vi "Harvest_Global.vi"() -> ()   [LabVIEW 2015]
panel:
  in  "stop":bool
  in  "Files pulled from Public":i32
  in  "Files Copied fr Server to Public":i32
  in  "Files copied fr Local to Public":i32
  in  "No Files to Pull":i32
  in  "Files pushed onto Server":i32
  in  "Done Transfer?":bool
  in  "No Files to Push":i32
  in  "File being transfered":path
  in  "Currently":string
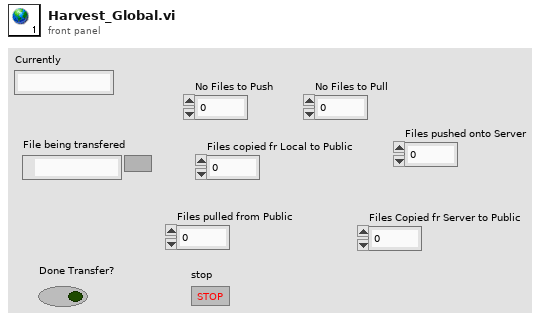
[diagram p1: front panel]
diagram:
